vi "Listen For Clients.vi"(8 "connection IDs In":refnum<k5>[](array[refnum]), 11 "listener ID in":refnum<k5>) -> (0 "connection IDs Out":refnum<k5>[](array[refnum]), 3 "listener ID out":refnum<k5>)   [LabVIEW 2018, in "Labview Python.lvlib"]
uses:
  Labview Python.lvlib
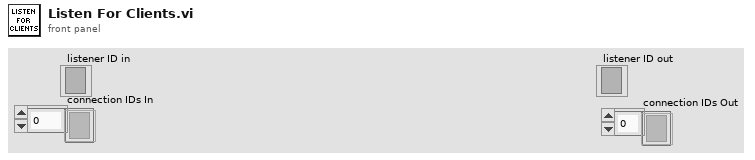
[diagram p1: front panel]
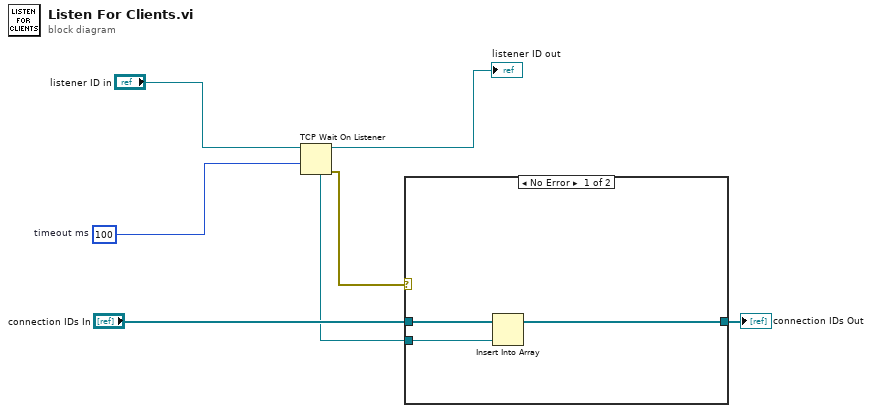
[diagram p0: block diagram]
diagram:
  w7 = 100  # timeout ms
  n1 = TCP Wait On Listener(9:w7, 11:"listener ID in") -> (0:w4:errorcluster, 3:→"listener ID out":refnum<k5>, 4:w2:refnum<k5>)  [unwired: 1 in, 3 out]
  n2 = case shown="No Error" w4 {
    tunnel: "connection IDs In" -> [w10 w11]
    tunnel: w2 -> [w9 _]
    tunnel: [w8 w11] -> w1
    frame No Error {
      n3 = Insert Into Array(array=w10, new element=w9) -> (w8:refnum<k5>[])  [unwired: 1 in]
    }
    frame Error {
    }
  }
  "connection IDs Out" <- w1
